vi "Transform coordinates.vi"(8 "Transform":T1, 10 "Y axis coordinate in":dbl, 11 "X axis coordinate in":dbl) -> (2 "New Y":dbl, 3 "New X":dbl)   [LabVIEW 2019]
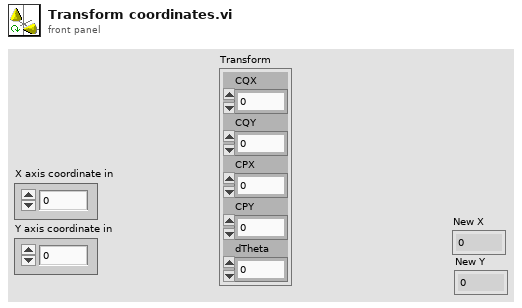
[diagram p1: front panel]
types:
  T1 = cluster{"CQX":dbl, "CQY":dbl, "CPX":dbl, "CPY":dbl, "dTheta":dbl}
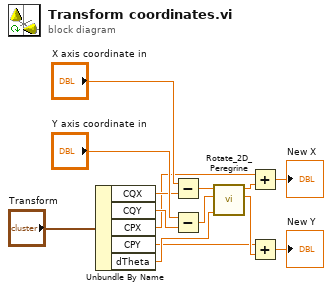
[diagram p0: block diagram]
diagram:
  n1 = Unbundle By Name("Transform") -> ("CQX"=w10:dbl, "CQY"=w12:dbl, "CPX"=w6:dbl, "CPY"=w3:dbl, "dTheta"=w7:dbl)
  n2 = Subtract(x="X axis coordinate in", y=w10) -> (x-y=w8:dbl)
  n3 = Subtract(x="Y axis coordinate in", y=w12) -> (x-y=w9:dbl)
  n4 = call "Rotate_2D_Peregrine.vi"("Angle(rad)"=w7, "Y axis coordinate in"=w9, "X axis coordinate in"=w8) -> ("Y axis coordinate out"=w4:dbl, "X axis coordinate out"=w5:dbl)  [unwired: 7 in]
  n5 = Add(x=w6, y=w5) -> (x+y=→"New X":dbl)
  n6 = Add(x=w3, y=w4) -> (x+y=→"New Y":dbl)
